vi "Fit.vi"(8 "error in (no error)":errorcluster caption="entrée d'erreur (pas d'erreur)", 9 "doc":string, 10 "raw_documents":string[][](array[string]), 11 "CountVectorizer.lvclass":refnum<class "CountVectorizer.lvclass">) -> (0 "error out":errorcluster caption="sortie d'erreur", 2 "String Data":string, 3 "CountVectorizer.lvclass":refnum<class "CountVectorizer.lvclass">)   [LabVIEW 2020, in "CountVectorizer.lvclass"]
doc: "Learn a vocabulary dictionary of all tokens in the raw documents.\n\nReturns :\n\n- String : OK"
uses:
  CountVectorizer.lvclass
  CountVectorizer.lvclass/CountVectorizer.ctl
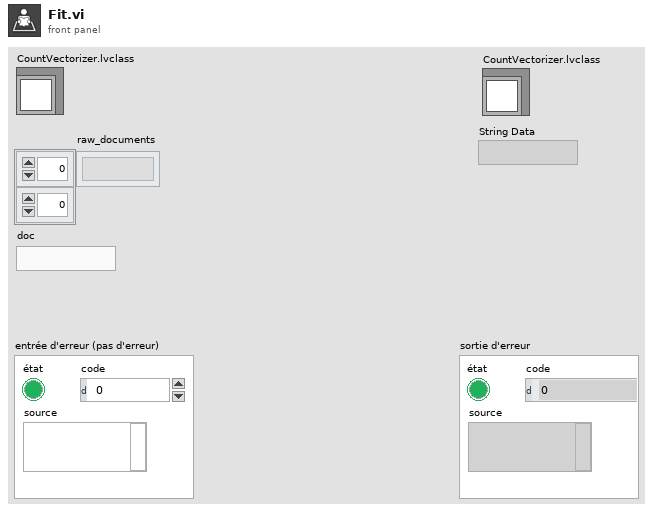
[diagram p1: front panel]
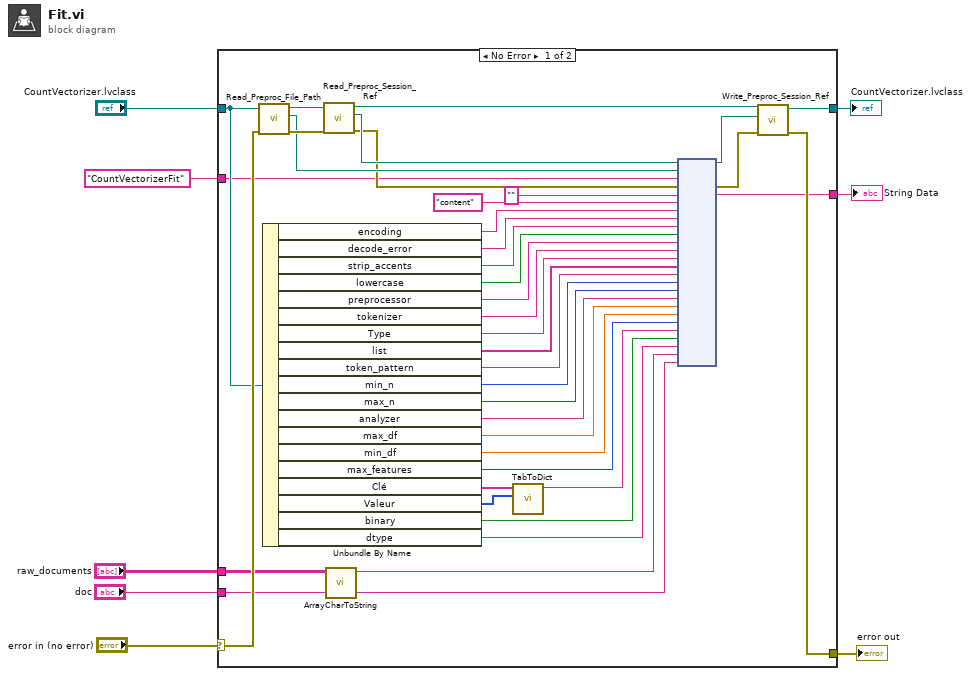
[diagram p0: block diagram]
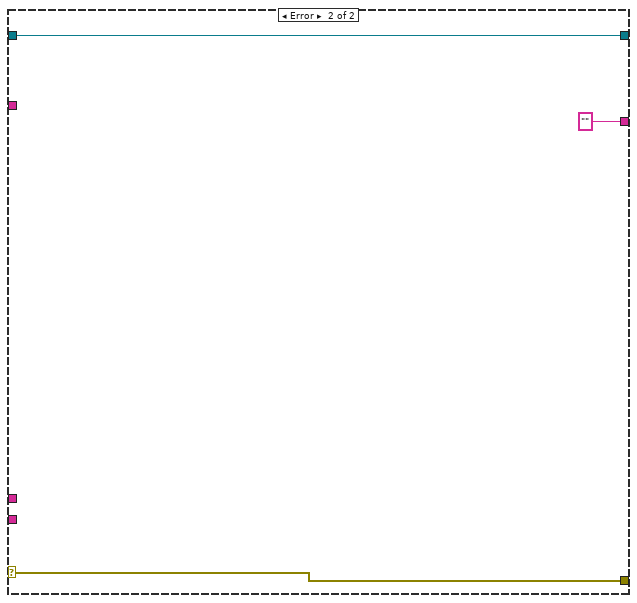
[diagram p2: hidden frame]
diagram:
  n1 = case shown="No Error" "error in (no error)" {
    selector: "error in (no error)" -> [w34 w50]
    tunnel: [w35 w50] -> w7
    tunnel: [w36 w49] -> w5
    tunnel: "CountVectorizer.lvclass" -> [w33 w49]
    tunnel: "CountVectorizerFit" ("Fonction") -> [w32 _]
    tunnel: [w31 ""] -> w3
    tunnel: "raw_documents" -> [w10 _]
    tunnel: "doc" -> [w11 _]
    frame No Error {
      n2 = call-dynamic "Read_Preproc_File_Path.vi"("error in (no error)"=w34, "Python in"=w33) -> ("error out"=w46:errorcluster, "File_Path"=w45:path, "Python out"=w47:refnum<class "CountVectorizer.lvclass">)  [unwired: 7 in]
      n3 = Unbundle By Name(w33) -> ("encoding"=w38:string, "decode_error"=w37:string, "strip_accents"=w30:string, "lowercase"=w29:bool, "preprocessor"=w28:string, "tokenizer"=w27:string, "Type"=w26:string, "list"=w22:string[], "token_pattern"=w21:string, "min_n"=w20:i32, "max_n"=w19:i32, "analyzer"=w18:string, "max_df"=w17:dbl, "min_df"=w16:dbl, "max_features"=w15:i32, "Clé"=w24:string[], "Valeur"=w23:i32[], "binary"=w13:bool, "dtype"=w12:string)
      n4 = call-dynamic "Read_Preproc_Session_Ref.vi"("error in (no error)"=w46, "Python in"=w47) -> ("error out"=w43:errorcluster, "Session_ref"=w44:refnum<k35>, "Python out"=w42:refnum<class "CountVectorizer.lvclass">)  [unwired: 7 in]
      n5 = call "ArrayCharToString.vi"("TAB"=w10) -> ("Instruction"=w9:string)  [unwired: 10 in]
      n6 = call "TabToDict.vi"("Int Value"=w23, "String key"=w24) -> ("Dict with int value"=w14:string)  [unwired: 8 in, 1 out]
      n7 = node(w44, w45, w32, w43, "", "content", w38, w37, w30, w29, w28, w27, w26, w22, w21, w20, w19, w18, w17, w16, w15, w14, w13, w12, w9, w11) -> (w40:refnum<k35>, w41:errorcluster, w31:string)  [unwired: 21 in, 2 out]
      n8 = call-dynamic "Write_Preproc_Session_Ref.vi"("error in (no error)"=w41, "Session_ref"=w40, "Python in"=w42) -> ("error out"=w35:errorcluster, "Python out"=w36:refnum<class "CountVectorizer.lvclass">)  [unwired: 7 in]
    }
    frame Error {
    }
  }
  "error out" <- w7
  "CountVectorizer.lvclass" <- w5
  "String Data" <- w3
